vi "init.vi"(0 "Constant Analog Output Voltage Test in":refnum<class "Constant Current Output Test.lvclass">, 1 "DAQ Channel 1":refnum<k21>, 2 "Expected Value":dbl format="%.3f", 3 "Tolerance":dbl format="%.3f", 4 "Samples To Average":i32, 5 "error in (no error)":errorcluster, 6 "DAQ Channel 2":refnum<k21>, 7 "Log":refnum<class "ITestLog.lvclass">, 8 "Test Scenario":T1, 9 "Resistance":dbl format="%.3f", 10 "Signal Name":string) -> (14 "Constant Analog Output Voltage Test  out":refnum<class "Constant Current Output Test.lvclass">, 19 "error out":errorcluster)   [LabVIEW 2015, in "Constant Current Output Test.lvclass"]
uses:
  Constant Current Output Test.lvclass
  Model/TestLog/ITestLog/ITestLog.lvclass
  Typedefs/TestScenarioTypes.ctl
  Constant Current Output Test.lvclass/Constant Current Output Test.ctl
  Typedefs/ILCBTTypedefs.lvlib
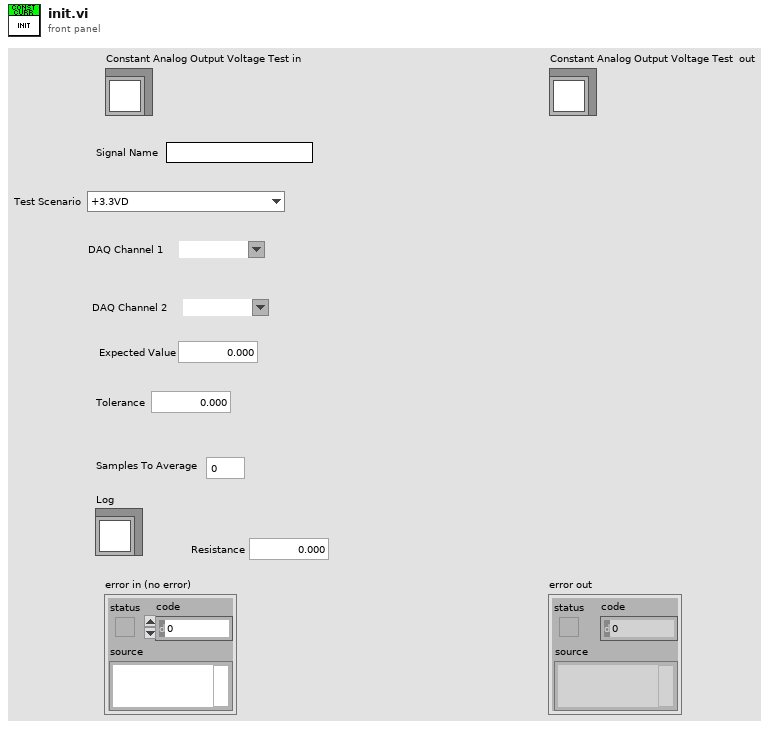
[diagram p1: front panel]
types:
  T1 = typedef "ILCBTTypedefs.lvlib/TestScenarioTypes.ctl" = enum16{"+3.3VD", "+5.1V", "+24V", "RELVALV1", "RELVALV2", "Verify DAC_A = -1.00A", "Verify DAC_A = -0.75A", "Verify DAC_A = -0.50A", "Verify DAC_A = -0.25A", "Verify DAC_A = 0.00A", "Verify DAC_A = 0.25A", "Verify DAC_A = 0.50A", "Verify DAC_A = 0.75A", "Verify DAC_A = 1.00A", "Verify DAC_B = -1.00A", "Verify DAC_B = -0.75A", "Verify DAC_B = -0.50A", "Verify DAC_B = -0.25A", "Verify DAC_B = 0.00A", "Verify DAC_B = 0.25A", "Verify DAC_B = 0.50A", "Verify DAC_B = 0.75A", "Verify DAC_B = 1.00A"}
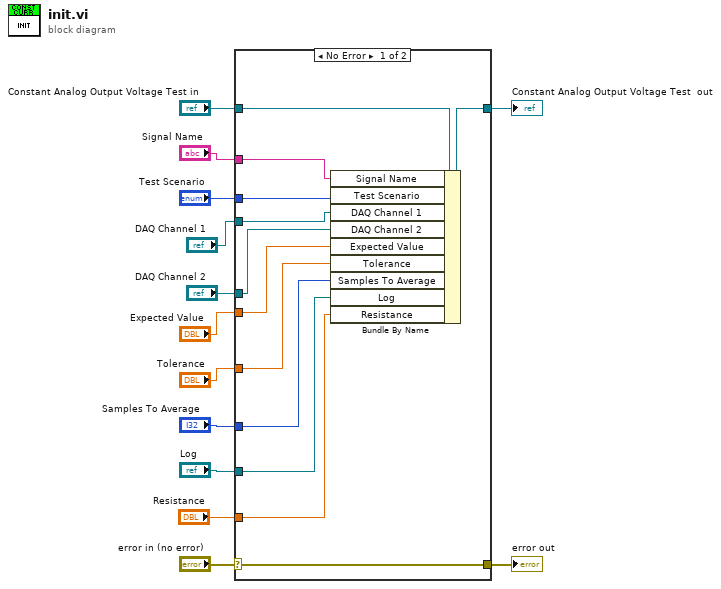
[diagram p0: block diagram]
diagram:
  n1 = case shown="No Error" "error in (no error)" {
    selector: "error in (no error)" -> [w25 w27]
    tunnel: [w25 w27] -> w12
    tunnel: [w23 w26] -> w10
    tunnel: "Constant Analog Output Voltage Test in" -> [w24 w26]
    tunnel: "DAQ Channel 1" -> [w16 _]
    tunnel: "Expected Value" -> [w22 _]
    tunnel: "Tolerance" -> [w21 _]
    tunnel: "Samples To Average" -> [w20 _]
    tunnel: "Log" -> [w19 _]
    tunnel: "Signal Name" -> [w18 _]
    tunnel: "Test Scenario" -> [w17 _]
    tunnel: "DAQ Channel 2" -> [w15 _]
    tunnel: "Resistance" -> [w14 _]
    frame No Error {
      n2 = Bundle By Name(cluster=w24, "Signal Name"=w18, "Test Scenario"=w17, "DAQ Channel 1"=w16, "DAQ Channel 2"=w15, "Expected Value"=w22, "Tolerance"=w21, "Samples To Average"=w20, "Log"=w19, "Resistance"=w14) -> (w23:refnum<class "Constant Current Output Test.lvclass">)
    }
    frame Error {
    }
  }
  "error out" <- w12
  "Constant Analog Output Voltage Test  out" <- w10
